vi "输入数据解析.vi"(0 "单个参数补充":dbl, 1 "从板号":dbl=1.0, 2 "主板二维码":string="BNET01", 3 "从板二维码":string="BNET01", 5 "主板引用":refnum<vi>, 7 "从板引用":refnum<vi>, 9 "主板选项":string="三级故障阀值", 11 "枚举":enum16{"主板", "从板"}(ring), 12 "快换":bool caption="快换写入") -> (4 "输出数组":dbl[][](array[numeric]), 6 "数组长度":dbl[](array[numeric]), 8 "循环次数":i32, 10 "命令":u32, 14 "名称":string[](array[string]), 15 "命令序号":u32[](array[numeric]))   [LabVIEW 2013] (continued)
                n681 = Build Array(w1614) -> (w1613:i32[])
              }
              frame 12 {
                # "SOC过高"
                n682 = Unbundle By Name(w1626) -> ("SOC过高"=w1625:dbl)
                n683 = call "输入分辨率计算-EV05.vi"("1字节?"=FALSE, "数值"=w1625, "偏移量"=0.0, "分辨率"=0.1) -> ("低字节"=w1627:dbl, "高字节1"=w1628:dbl)  [unwired: 1 in, 5 out]
                n684 = call "二进制解析-8.6.vi"("索引"=4, "数值"=w1628) -> ("低位子数组"=w1631:i32[])  [unwired: 3 out]
                n685 = call "二进制解析-8.6.vi"("索引"=4, "数值"=w1627) -> ("低位子数组"=w1623:i32[], "高位子数组"=w1630:i32[])  [unwired: 2 out]
                n686 = Insert Into Array(array=w1631, new element=w1630) -> (w1629:i32[])  [unwired: 1 in]
                n687 = call "数值二进制转十进制-8.6.vi"("子数组"=w1629) -> ("十进制数值"=w1624:i32)  [unwired: 4 out]
                n688 = disable-structure shown="启用" {
                  disable-tunnel: w1624 -> [w1639 _]
                  disable-tunnel: [w1639 255 ("高字节1")] -> w1622
                  disable-tunnel: [w1638 i32[] [] ("低位子数组 20")] -> _
                  disable-tunnel: w1623 -> [w1638 _]
                  frame Disabled {
                  }
                  frame Enabled {
                  }
                }
                n689 = Build Array(w1622, w1622) -> (w1635:i32[])
              }
              frame 13 {
                # "SOC过低"
                n690 = Unbundle By Name(w1648) -> ("SOC过低"=w1647:dbl)
                n691 = call "输入分辨率计算-EV05.vi"("1字节?"=FALSE, "数值"=w1647, "偏移量"=0.0, "分辨率"=0.1) -> ("低字节"=w1645:dbl, "高字节1"=w1646:dbl)  [unwired: 1 in, 5 out]
                n692 = call "二进制解析-8.6.vi"("索引"=4, "数值"=w1646) -> ("低位子数组"=w1643:i32[])  [unwired: 3 out]
                n693 = disable-structure shown="启用" {
                  disable-tunnel: w1645 -> [w1655 _]
                  disable-tunnel: [w1655 255 ("高字节1")] -> w1644
                  disable-tunnel: w1643 -> [w1654 _]
                  disable-tunnel: [_ 255 ("高字节1")] -> w1642
                  frame Disabled {
                    (unwired) i32[] [] ("低位子数组 4")
                  }
                  frame Enabled {
                  }
                }
                n694 = Build Array(w1642, w1644) -> (w1651:i32[])
              }
              frame 14 {
                # "内阻过大"
                n695 = disable-structure shown="启用" {
                  disable-tunnel: w1660 -> [w1665 _]
                  disable-tunnel: [w1661 255 ("高字节1")] -> w1658
                  frame Disabled {
                    n696 = Unbundle By Name(w1665) -> ("内阻过大"=w1664:dbl)
                    n697 = call "输入分辨率计算-EV05.vi"("1字节?"=TRUE, "数值"=w1664, "分辨率"=0.1) -> ("高字节1"=w1661:dbl)  [unwired: 2 in, 6 out]
                  }
                  frame Enabled {
                  }
                }
                n698 = Build Array(w1658) -> (w1659:i32[])
              }
              frame 15 {
                # "极柱温度过高"
                n699 = disable-structure shown="启用" {
                  disable-tunnel: w1669 -> [w1675 _]
                  disable-tunnel: [w1671 255 ("高字节1")] -> w1667
                  frame Disabled {
                    n700 = Unbundle By Name(w1675) -> ("极柱温度过高"=w1674:dbl)
                    n701 = call "输入分辨率计算-EV05.vi"("1字节?"=TRUE, "数值"=w1674, "偏移量"=-40.0, "分辨率"=1.0) -> ("高字节1"=w1671:dbl)  [unwired: 1 in, 6 out]
                  }
                  frame Enabled {
                  }
                }
                n702 = Build Array(w1667) -> (w1668:i32[])
              }
              frame 16 {
                # "SOH过低"
                n703 = disable-structure shown="启用" {
                  disable-tunnel: [w1692 w1700] -> w1679
                  disable-tunnel: w1678 -> [w1689 _]
                  disable-tunnel: [w1681 w1700] -> w1677
                  frame Disabled {
                    n704 = Unbundle By Name(w1689) -> ("SOH过低"=w1688:dbl)
                    n705 = call "输入分辨率计算-EV05.vi"("1字节?"=FALSE, "数值"=w1688, "偏移量"=0.0, "分辨率"=0.1) -> ("低字节"=w1690:dbl, "高字节1"=w1691:dbl)  [unwired: 1 in, 5 out]
                    n706 = call "二进制解析-8.6.vi"("索引"=4, "数值"=w1691) -> ("低位子数组"=w1694:i32[])  [unwired: 3 out]
                    n707 = call "二进制解析-8.6.vi"("索引"=4, "数值"=w1690) -> ("低位子数组"=w1683:i32[], "高位子数组"=w1693:i32[])  [unwired: 2 out]
                    n708 = call "二进制解析-8.6.vi"("索引"=4, "数值"=0) -> ("低位子数组"=w1684:i32[])  [unwired: 3 out]
                    n709 = Insert Into Array(array=w1694, new element=w1693) -> (w1687:i32[])  [unwired: 1 in]
                    n710 = Insert Into Array(array=w1683, new element=w1684) -> (w1682:i32[])  [unwired: 1 in]
                    n711 = call "数值二进制转十进制-8.6.vi"("子数组"=w1687) -> ("十进制数值"=w1692:i32)  [unwired: 4 out]
                    n712 = call "数值二进制转十进制-8.6.vi"("子数组"=w1682) -> ("十进制数值"=w1681:i32)  [unwired: 4 out]
                  }
                  frame Enabled {
                    w1700 = 255 ("高字节1")
                  }
                }
                n713 = Build Array(w1679, w1677) -> (w1680:i32[])
              }
            }
            n714 = Insert Into Array(array=w1484, new element=w1485) -> (w1483:dbl[])  [unwired: 1 in]
          }
          n715 = Build Array(w1480) -> (w1479:dbl[][])
          n716 = Build Array("一级故障阀值") -> (w1470:string[])
        }
        frame "总电压过低(2)" {
          n717 = Unbundle By Name(w1706) -> ("一级故障 2"=w1707:refnum<vi>)
          n718 = property class="Clust (严格)"(reference=w1707) -> ("Value"=w1705:T4)  [unwired: 1 in, 2 out]
          n719 = for {
            N: 17 -> [_]
            tunnel: w1705 -> [w1717]
            shift-right: [w1714] -> w1711
            shift-left: dbl[] [] -> [w1715]
            i -> [w1718]
            n720 = case shown="13" w1718 {
              tunnel: w1717 -> [w1719 w1730 w1741 w1751 w1761 w1771 w1783 w1795 w1807 w1819 w1831 w1843 w1857 w1879 w1891 w1900 w1909]
              tunnel: [w1720 w1731 w1742 w1752 w1762 w1773 w1785 w1797 w1809 w1821 w1833 w1844 w1866 w1882 w1890 w1899 w1911] -> w1716
              frame 0, Default {
                # "总电压过高"
                n721 = disable-structure shown="启用" {
                  disable-tunnel: [w1726 w1729] -> w1722
                  disable-tunnel: [w1725 w1729] -> w1721
                  disable-tunnel: w1719 -> [w1724 _]
                  frame Disabled {
                    n722 = Unbundle By Name(w1724) -> ("总电压过高"=w1723:dbl)
                    n723 = call "输入分辨率计算-EV05.vi"("1字节?"=FALSE, "数值"=w1723, "分辨率"=0.1) -> ("低字节"=w1726:dbl, "高字节1"=w1725:dbl)  [unwired: 2 in, 5 out]
                  }
                  frame Enabled {
                    w1729 = 255 ("高字节1")
                  }
                }
                n724 = Build Array(w1721, w1722) -> (w1720:i32[])
              }
              frame 1 {
                # "总电压过低"
                n725 = disable-structure shown="启用" {
                  disable-tunnel: [w1737 w1740] -> w1733
                  disable-tunnel: [w1736 w1740] -> w1732
                  disable-tunnel: w1730 -> [w1735 _]
                  frame Enabled {
                    n726 = Unbundle By Name(w1735) -> ("总电压过低"=w1734:dbl)
                    n727 = call "输入分辨率计算-EV05.vi"("1字节?"=FALSE, "数值"=w1734, "分辨率"=0.1) -> ("低字节"=w1737:dbl, "高字节1"=w1736:dbl)  [unwired: 2 in, 5 out]
                  }
                  frame Disabled {
                    w1740 = 255 ("高字节1")
                  }
                }
                n728 = Build Array(w1732, w1733) -> (w1731:dbl[])
              }
              frame 2 {
                # "温度过高"
                n729 = disable-structure shown="启用" {
                  disable-tunnel: [w1747 255 ("高字节1")] -> w1743
                  disable-tunnel: w1741 -> [w1745 _]
                  frame Disabled {
                    n730 = Unbundle By Name(w1745) -> ("温度过高"=w1744:dbl)
                    n731 = call "输入分辨率计算-EV05.vi"("1字节?"=TRUE, "数值"=w1744, "偏移量"=-40.0, "分辨率"=1.0) -> ("高字节1"=w1747:dbl)  [unwired: 1 in, 6 out]
                  }
                  frame Enabled {
                  }
                }
                n732 = Build Array(w1743) -> (w1742:i32[])
              }
              frame 3 {
                # "温度过低"
                n733 = disable-structure shown="启用" {
                  disable-tunnel: [w1757 255 ("高字节1")] -> w1753
                  disable-tunnel: w1751 -> [w1755 _]
                  frame Disabled {
                    n734 = Unbundle By Name(w1755) -> ("温度过低"=w1754:dbl)
                    n735 = call "输入分辨率计算-EV05.vi"("1字节?"=TRUE, "数值"=w1754, "偏移量"=-40.0, "分辨率"=1.0) -> ("高字节1"=w1757:dbl)  [unwired: 1 in, 6 out]
                  }
                  frame Enabled {
                  }
                }
                n736 = Build Array(w1753) -> (w1752:i32[])
              }
              frame 4 {
                # "整组温度不均衡"
                n737 = disable-structure shown="启用" {
                  disable-tunnel: [w1767 255 ("高字节1")] -> w1763
                  disable-tunnel: w1761 -> [w1765 _]
                  frame Disabled {
                    n738 = Unbundle By Name(w1765) -> ("整组温度不均衡"=w1764:dbl)
                    n739 = call "输入分辨率计算-EV05.vi"("1字节?"=TRUE, "数值"=w1764, "偏移量"=0.0, "分辨率"=1.0) -> ("高字节1"=w1767:dbl)  [unwired: 1 in, 6 out]
                  }
                  frame Enabled {
                  }
                }
                n740 = Build Array(w1763) -> (w1762:i32[])
              }
              frame 5 {
                # "单组电压不均衡"
                n741 = disable-structure shown="启用" {
                  disable-tunnel: [w1779 w1782] -> w1774
                  disable-tunnel: [w1777 w1782] -> w1772
                  disable-tunnel: w1771 -> [w1776 _]
                  frame Disabled {
                    n742 = Unbundle By Name(w1776) -> ("单组电压不均衡"=w1775:dbl)
                    n743 = call "输入分辨率计算-EV05.vi"("1字节?"=FALSE, "数值"=w1775, "偏移量"=0.0, "分辨率"=0.001) -> ("低字节"=w1777:dbl, "高字节1"=w1779:dbl)  [unwired: 1 in, 5 out]
                  }
                  frame Enabled {
                    w1782 = 255 ("高字节1")
                  }
                }
                n744 = Build Array(w1774, w1772) -> (w1773:i32[])
              }
              frame 6 {
                # "整组电压不均衡"
                n745 = disable-structure shown="启用" {
                  disable-tunnel: [w1791 w1794] -> w1786
                  disable-tunnel: [w1789 w1794] -> w1784
                  disable-tunnel: w1783 -> [w1788 _]
                  frame Disabled {
                    n746 = Unbundle By Name(w1788) -> ("整组电压不均衡"=w1787:dbl)
                    n747 = call "输入分辨率计算-EV05.vi"("1字节?"=FALSE, "数值"=w1787, "偏移量"=0.0, "分辨率"=0.001) -> ("低字节"=w1789:dbl, "高字节1"=w1791:dbl)  [unwired: 1 in, 5 out]
                  }
                  frame Enabled {
                    w1794 = 255 ("高字节1")
                  }
                }
                n748 = Build Array(w1786, w1784) -> (w1785:i32[])
              }
              frame 7 {
                # "单体电压过高"
                n749 = disable-structure shown="启用" {
                  disable-tunnel: [w1803 w1806] -> w1798
                  disable-tunnel: [w1801 w1806] -> w1796
                  disable-tunnel: w1795 -> [w1800 _]
                  frame Disabled {
                    n750 = Unbundle By Name(w1800) -> ("单体电压过高"=w1799:dbl)
                    n751 = call "输入分辨率计算-EV05.vi"("1字节?"=FALSE, "数值"=w1799, "偏移量"=0.0, "分辨率"=0.001) -> ("低字节"=w1801:dbl, "高字节1"=w1803:dbl)  [unwired: 1 in, 5 out]
                  }
                  frame Enabled {
                    w1806 = 255 ("高字节1")
                  }
                }
                n752 = Build Array(w1798, w1796) -> (w1797:i32[])
              }
              frame 8 {
                # "单体电压过低"
                n753 = disable-structure shown="启用" {
                  disable-tunnel: [w1815 w1818] -> w1810
                  disable-tunnel: [w1813 w1818] -> w1808
                  disable-tunnel: w1807 -> [w1812 _]
                  frame Disabled {
                    n754 = Unbundle By Name(w1812) -> ("单体电压过低"=w1811:dbl)
                    n755 = call "输入分辨率计算-EV05.vi"("1字节?"=FALSE, "数值"=w1811, "偏移量"=0.0, "分辨率"=0.001) -> ("低字节"=w1813:dbl, "高字节1"=w1815:dbl)  [unwired: 1 in, 5 out]
                  }
                  frame Enabled {
                    w1818 = 255 ("高字节1")
                  }
                }
                n756 = Build Array(w1810, w1808) -> (w1809:i32[])
              }
              frame 9 {
                # "充电电流过高"
                n757 = disable-structure shown="启用" {
                  disable-tunnel: [w1827 w1830] -> w1822
                  disable-tunnel: [w1825 w1830] -> w1820
                  disable-tunnel: w1819 -> [w1824 _]
                  frame Disabled {
                    n758 = Unbundle By Name(w1824) -> ("充电电流过高"=w1823:dbl)
                    n759 = call "输入分辨率计算-EV05.vi"("1字节?"=FALSE, "数值"=w1823, "偏移量"=-3000.0, "分辨率"=0.1) -> ("低字节"=w1825:dbl, "高字节1"=w1827:dbl)  [unwired: 1 in, 5 out]
                  }
                  frame Enabled {
                    w1830 = 255 ("高字节1")
                  }
                }
                n760 = Build Array(w1822, w1820) -> (w1821:i32[])
              }
              frame 10 {
                # "放电电流过高"
                n761 = disable-structure shown="启用" {
                  disable-tunnel: [w1839 w1842] -> w1834
                  disable-tunnel: [w1837 w1842] -> w1832
                  disable-tunnel: w1831 -> [w1836 _]
                  frame Disabled {
                    n762 = Unbundle By Name(w1836) -> ("放电电流过高"=w1835:dbl)
                    n763 = call "输入分辨率计算-EV05.vi"("1字节?"=FALSE, "数值"=w1835, "偏移量"=-3000.0, "分辨率"=0.1) -> ("低字节"=w1837:dbl, "高字节1"=w1839:dbl)  [unwired: 1 in, 5 out]
                  }
                  frame Enabled {
                    w1842 = 255 ("高字节1")
                  }
                }
                n764 = Build Array(w1834, w1832) -> (w1833:i32[])
              }
              frame 11 {
                # "单组温度不均衡"
                n765 = disable-structure shown="启用" {
                  disable-tunnel: [w1849 255 ("高字节1")] -> w1845
                  disable-tunnel: w1843 -> [w1847 _]
                  frame Disabled {
                    n766 = Unbundle By Name(w1847) -> ("单组温度不均衡"=w1846:dbl)
                    n767 = call "输入分辨率计算-EV05.vi"("1字节?"=TRUE, "数值"=w1846, "偏移量"=0.0, "分辨率"=1.0) -> ("高字节1"=w1849:dbl)  [unwired: 1 in, 6 out]
                  }
                  frame Enabled {
                  }
                }
                n768 = Build Array(w1845) -> (w1844:i32[])
              }
              frame 12 {
                # "SOC过高"
                n769 = Unbundle By Name(w1857) -> ("SOC过高"=w1856:dbl)
                n770 = call "输入分辨率计算-EV05.vi"("1字节?"=FALSE, "数值"=w1856, "偏移量"=0.0, "分辨率"=0.1) -> ("低字节"=w1858:dbl, "高字节1"=w1859:dbl)  [unwired: 1 in, 5 out]
                n771 = call "二进制解析-8.6.vi"("索引"=4, "数值"=w1859) -> ("低位子数组"=w1862:i32[])  [unwired: 3 out]
                n772 = call "二进制解析-8.6.vi"("索引"=4, "数值"=w1858) -> ("低位子数组"=w1854:i32[], "高位子数组"=w1861:i32[])  [unwired: 2 out]
                n773 = Insert Into Array(array=w1862, new element=w1861) -> (w1860:i32[])  [unwired: 1 in]
                n774 = call "数值二进制转十进制-8.6.vi"("子数组"=w1860) -> ("十进制数值"=w1855:i32)  [unwired: 4 out]
                n775 = disable-structure shown="启用" {
                  disable-tunnel: w1855 -> [w1870 _]
                  disable-tunnel: [w1870 255 ("高字节1")] -> w1853
                  disable-tunnel: [w1869 i32[] [] ("低位子数组 20")] -> _
                  disable-tunnel: w1854 -> [w1869 _]
                  frame Disabled {
                  }
                  frame Enabled {
                  }
                }
                n776 = Build Array(w1853, w1853) -> (w1866:i32[])
              }
              frame 13 {
                # "SOC过低"
                n777 = Unbundle By Name(w1879) -> ("SOC过低"=w1878:dbl)
                n778 = call "输入分辨率计算-EV05.vi"("1字节?"=FALSE, "数值"=w1878, "偏移量"=0.0, "分辨率"=0.1) -> ("低字节"=w1876:dbl, "高字节1"=w1877:dbl)  [unwired: 1 in, 5 out]
                n779 = call "二进制解析-8.6.vi"("索引"=4, "数值"=w1877) -> ("低位子数组"=w1874:i32[])  [unwired: 3 out]
                n780 = disable-structure shown="启用" {
                  disable-tunnel: w1876 -> [w1886 _]
                  disable-tunnel: [w1886 255 ("高字节1")] -> w1875
                  disable-tunnel: w1874 -> [w1885 _]
                  disable-tunnel: [_ 255 ("高字节1")] -> w1873
                  frame Disabled {
                    (unwired) i32[] [] ("低位子数组 4")
                  }
                  frame Enabled {
                  }
                }
                n781 = Build Array(w1873, w1875) -> (w1882:i32[])
              }
              frame 14 {
                # "内阻过大"
                n782 = disable-structure shown="启用" {
                  disable-tunnel: w1891 -> [w1896 _]
                  disable-tunnel: [w1892 255 ("高字节1")] -> w1889
                  frame Disabled {
                    n783 = Unbundle By Name(w1896) -> ("内阻过大"=w1895:dbl)
                    n784 = call "输入分辨率计算-EV05.vi"("1字节?"=TRUE, "数值"=w1895, "分辨率"=0.1) -> ("高字节1"=w1892:dbl)  [unwired: 2 in, 6 out]
                  }
                  frame Enabled {
                  }
                }
                n785 = Build Array(w1889) -> (w1890:i32[])
              }
              frame 15 {
                # "极柱温度过高"
                n786 = disable-structure shown="启用" {
                  disable-tunnel: w1900 -> [w1906 _]
                  disable-tunnel: [w1902 255 ("高字节1")] -> w1898
                  frame Disabled {
                    n787 = Unbundle By Name(w1906) -> ("极柱温度过高"=w1905:dbl)
                    n788 = call "输入分辨率计算-EV05.vi"("1字节?"=TRUE, "数值"=w1905, "偏移量"=-40.0, "分辨率"=1.0) -> ("高字节1"=w1902:dbl)  [unwired: 1 in, 6 out]
                  }
                  frame Enabled {
                  }
                }
                n789 = Build Array(w1898) -> (w1899:i32[])
              }
              frame 16 {
                # "SOH过低"
                n790 = disable-structure shown="启用" {
                  disable-tunnel: [w1923 w1931] -> w1910
                  disable-tunnel: w1909 -> [w1920 _]
                  disable-tunnel: [w1912 w1931] -> w1908
                  frame Disabled {
                    n791 = Unbundle By Name(w1920) -> ("SOH过低"=w1919:dbl)
                    n792 = call "输入分辨率计算-EV05.vi"("1字节?"=FALSE, "数值"=w1919, "偏移量"=0.0, "分辨率"=0.1) -> ("低字节"=w1921:dbl, "高字节1"=w1922:dbl)  [unwired: 1 in, 5 out]
                    n793 = call "二进制解析-8.6.vi"("索引"=4, "数值"=w1922) -> ("低位子数组"=w1925:i32[])  [unwired: 3 out]
                    n794 = call "二进制解析-8.6.vi"("索引"=4, "数值"=w1921) -> ("低位子数组"=w1914:i32[], "高位子数组"=w1924:i32[])  [unwired: 2 out]
                    n795 = call "二进制解析-8.6.vi"("索引"=4, "数值"=0) -> ("低位子数组"=w1915:i32[])  [unwired: 3 out]
                    n796 = Insert Into Array(array=w1925, new element=w1924) -> (w1918:i32[])  [unwired: 1 in]
                    n797 = Insert Into Array(array=w1914, new element=w1915) -> (w1913:i32[])  [unwired: 1 in]
                    n798 = call "数值二进制转十进制-8.6.vi"("子数组"=w1918) -> ("十进制数值"=w1923:i32)  [unwired: 4 out]
                    n799 = call "数值二进制转十进制-8.6.vi"("子数组"=w1913) -> ("十进制数值"=w1912:i32)  [unwired: 4 out]
                  }
                  frame Enabled {
                    w1931 = 255 ("高字节1")
                  }
                }
                n800 = Build Array(w1910, w1908) -> (w1911:i32[])
              }
            }
            n801 = Insert Into Array(array=w1715, new element=w1716) -> (w1714:dbl[])  [unwired: 1 in]
          }
          n802 = Build Array(w1711) -> (w1710:dbl[][])
          n803 = Build Array("二级故障阀值") -> (w1701:string[])
        }
        frame "总电压过低(3)" {
          n804 = Unbundle By Name(w1937) -> ("一级故障 3"=w1938:refnum<vi>)
          n805 = property class="Clust (严格)"(reference=w1938) -> ("Value"=w1936:T4)  [unwired: 1 in, 2 out]
          n806 = for {
            N: 17 -> [_]
            tunnel: w1936 -> [w1948]
            shift-right: [w1945] -> w1942
            shift-left: dbl[] [] -> [w1946]
            i -> [w1949]
            n807 = case shown="13" w1949 {
              tunnel: w1948 -> [w1950 w1961 w1972 w1982 w1992 w2002 w2014 w2026 w2038 w2050 w2062 w2074 w2088 w2110 w2122 w2131 w2140]
              tunnel: [w1951 w1962 w1973 w1983 w1993 w2004 w2016 w2028 w2040 w2052 w2064 w2075 w2097 w2113 w2121 w2130 w2142] -> w1947
              frame 0, Default {
                # "总电压过高"
                n808 = disable-structure shown="启用" {
                  disable-tunnel: [w1957 w1960] -> w1953
                  disable-tunnel: [w1956 w1960] -> w1952
                  disable-tunnel: w1950 -> [w1955 _]
                  frame Disabled {
                    n809 = Unbundle By Name(w1955) -> ("总电压过高"=w1954:dbl)
                    n810 = call "输入分辨率计算-EV05.vi"("1字节?"=FALSE, "数值"=w1954, "分辨率"=0.1) -> ("低字节"=w1957:dbl, "高字节1"=w1956:dbl)  [unwired: 2 in, 5 out]
                  }
                  frame Enabled {
                    w1960 = 255 ("高字节1")
                  }
                }
                n811 = Build Array(w1952, w1953) -> (w1951:i32[])
              }
              frame 1 {
                # "总电压过低"
                n812 = disable-structure shown="启用" {
                  disable-tunnel: [w1968 w1971] -> w1964
                  disable-tunnel: [w1967 w1971] -> w1963
                  disable-tunnel: w1961 -> [w1966 _]
                  frame Enabled {
                    n813 = Unbundle By Name(w1966) -> ("总电压过低"=w1965:dbl)
                    n814 = call "输入分辨率计算-EV05.vi"("1字节?"=FALSE, "数值"=w1965, "分辨率"=0.1) -> ("低字节"=w1968:dbl, "高字节1"=w1967:dbl)  [unwired: 2 in, 5 out]
                  }
                  frame Disabled {
                    w1971 = 255 ("高字节1")
                  }
                }
                n815 = Build Array(w1963, w1964) -> (w1962:dbl[])
              }
              frame 2 {
                # "温度过高"
                n816 = disable-structure shown="启用" {
                  disable-tunnel: [w1978 255 ("高字节1")] -> w1974
                  disable-tunnel: w1972 -> [w1976 _]
                  frame Disabled {
                    n817 = Unbundle By Name(w1976) -> ("温度过高"=w1975:dbl)
                    n818 = call "输入分辨率计算-EV05.vi"("1字节?"=TRUE, "数值"=w1975, "偏移量"=-40.0, "分辨率"=1.0) -> ("高字节1"=w1978:dbl)  [unwired: 1 in, 6 out]
                  }
                  frame Enabled {
                  }
                }
                n819 = Build Array(w1974) -> (w1973:i32[])
              }
              frame 3 {
                # "温度过低"
                n820 = disable-structure shown="启用" {
                  disable-tunnel: [w1988 255 ("高字节1")] -> w1984
                  disable-tunnel: w1982 -> [w1986 _]
                  frame Disabled {
                    n821 = Unbundle By Name(w1986) -> ("温度过低"=w1985:dbl)
                    n822 = call "输入分辨率计算-EV05.vi"("1字节?"=TRUE, "数值"=w1985, "偏移量"=-40.0, "分辨率"=1.0) -> ("高字节1"=w1988:dbl)  [unwired: 1 in, 6 out]
                  }
                  frame Enabled {
                  }
                }
                n823 = Build Array(w1984) -> (w1983:i32[])
              }
              frame 4 {
                # "整组温度不均衡"
                n824 = disable-structure shown="启用" {
                  disable-tunnel: [w1998 255 ("高字节1")] -> w1994
                  disable-tunnel: w1992 -> [w1996 _]
                  frame Disabled {
                    n825 = Unbundle By Name(w1996) -> ("整组温度不均衡"=w1995:dbl)
                    n826 = call "输入分辨率计算-EV05.vi"("1字节?"=TRUE, "数值"=w1995, "偏移量"=0.0, "分辨率"=1.0) -> ("高字节1"=w1998:dbl)  [unwired: 1 in, 6 out]
                  }
                  frame Enabled {
                  }
                }
                n827 = Build Array(w1994) -> (w1993:i32[])
              }
              frame 5 {
                # "单组电压不均衡"
                n828 = disable-structure shown="启用" {
                  disable-tunnel: [w2010 w2013] -> w2005
                  disable-tunnel: [w2008 w2013] -> w2003
                  disable-tunnel: w2002 -> [w2007 _]
                  frame Disabled {
                    n829 = Unbundle By Name(w2007) -> ("单组电压不均衡"=w2006:dbl)
                    n830 = call "输入分辨率计算-EV05.vi"("1字节?"=FALSE, "数值"=w2006, "偏移量"=0.0, "分辨率"=0.001) -> ("低字节"=w2008:dbl, "高字节1"=w2010:dbl)  [unwired: 1 in, 5 out]
                  }
                  frame Enabled {
                    w2013 = 255 ("高字节1")
                  }
                }
                n831 = Build Array(w2005, w2003) -> (w2004:i32[])
              }
              frame 6 {
                # "整组电压不均衡"
                n832 = disable-structure shown="启用" {
                  disable-tunnel: [w2022 w2025] -> w2017
                  disable-tunnel: [w2020 w2025] -> w2015
                  disable-tunnel: w2014 -> [w2019 _]
                  frame Disabled {
                    n833 = Unbundle By Name(w2019) -> ("整组电压不均衡"=w2018:dbl)
                    n834 = call "输入分辨率计算-EV05.vi"("1字节?"=FALSE, "数值"=w2018, "偏移量"=0.0, "分辨率"=0.001) -> ("低字节"=w2020:dbl, "高字节1"=w2022:dbl)  [unwired: 1 in, 5 out]
                  }
                  frame Enabled {
                    w2025 = 255 ("高字节1")
                  }
                }
                n835 = Build Array(w2017, w2015) -> (w2016:i32[])
              }
              frame 7 {
                # "单体电压过高"
                n836 = disable-structure shown="启用" {
                  disable-tunnel: [w2034 w2037] -> w2029
                  disable-tunnel: [w2032 w2037] -> w2027
                  disable-tunnel: w2026 -> [w2031 _]
                  frame Disabled {
                    n837 = Unbundle By Name(w2031) -> ("单体电压过高"=w2030:dbl)
                    n838 = call "输入分辨率计算-EV05.vi"("1字节?"=FALSE, "数值"=w2030, "偏移量"=0.0, "分辨率"=0.001) -> ("低字节"=w2032:dbl, "高字节1"=w2034:dbl)  [unwired: 1 in, 5 out]
                  }
                  frame Enabled {
                    w2037 = 255 ("高字节1")
                  }
                }
                n839 = Build Array(w2029, w2027) -> (w2028:i32[])
              }
              frame 8 {
                # "单体电压过低"
                n840 = disable-structure shown="启用" {
                  disable-tunnel: [w2046 w2049] -> w2041
                  disable-tunnel: [w2044 w2049] -> w2039
                  disable-tunnel: w2038 -> [w2043 _]
                  frame Disabled {
                    n841 = Unbundle By Name(w2043) -> ("单体电压过低"=w2042:dbl)
                    n842 = call "输入分辨率计算-EV05.vi"("1字节?"=FALSE, "数值"=w2042, "偏移量"=0.0, "分辨率"=0.001) -> ("低字节"=w2044:dbl, "高字节1"=w2046:dbl)  [unwired: 1 in, 5 out]
                  }
                  frame Enabled {
                    w2049 = 255 ("高字节1")
                  }
                }
                n843 = Build Array(w2041, w2039) -> (w2040:i32[])
              }
              frame 9 {
                # "充电电流过高"
                n844 = disable-structure shown="启用" {
                  disable-tunnel: [w2058 w2061] -> w2053
                  disable-tunnel: [w2056 w2061] -> w2051
                  disable-tunnel: w2050 -> [w2055 _]
                  frame Disabled {
                    n845 = Unbundle By Name(w2055) -> ("充电电流过高"=w2054:dbl)
                    n846 = call "输入分辨率计算-EV05.vi"("1字节?"=FALSE, "数值"=w2054, "偏移量"=-3000.0, "分辨率"=0.1) -> ("低字节"=w2056:dbl, "高字节1"=w2058:dbl)  [unwired: 1 in, 5 out]
                  }
                  frame Enabled {
                    w2061 = 255 ("高字节1")
                  }
                }
                n847 = Build Array(w2053, w2051) -> (w2052:i32[])
              }
              frame 10 {
                # "放电电流过高"
                n848 = disable-structure shown="启用" {
                  disable-tunnel: [w2070 w2073] -> w2065
                  disable-tunnel: [w2068 w2073] -> w2063
                  disable-tunnel: w2062 -> [w2067 _]
                  frame Disabled {
                    n849 = Unbundle By Name(w2067) -> ("放电电流过高"=w2066:dbl)
                    n850 = call "输入分辨率计算-EV05.vi"("1字节?"=FALSE, "数值"=w2066, "偏移量"=-3000.0, "分辨率"=0.1) -> ("低字节"=w2068:dbl, "高字节1"=w2070:dbl)  [unwired: 1 in, 5 out]
                  }
                  frame Enabled {
                    w2073 = 255 ("高字节1")
                  }
                }
                n851 = Build Array(w2065, w2063) -> (w2064:i32[])
              }
              frame 11 {
                # "单组温度不均衡"
                n852 = disable-structure shown="启用" {
                  disable-tunnel: [w2080 255 ("高字节1")] -> w2076
                  disable-tunnel: w2074 -> [w2078 _]
                  frame Disabled {
                    n853 = Unbundle By Name(w2078) -> ("单组温度不均衡"=w2077:dbl)
                    n854 = call "输入分辨率计算-EV05.vi"("1字节?"=TRUE, "数值"=w2077, "偏移量"=0.0, "分辨率"=1.0) -> ("高字节1"=w2080:dbl)  [unwired: 1 in, 6 out]
                  }
                  frame Enabled {
                  }
                }
                n855 = Build Array(w2076) -> (w2075:i32[])
              }
              frame 12 {
                # "SOC过高"
                n856 = Unbundle By Name(w2088) -> ("SOC过高"=w2087:dbl)
                n857 = call "输入分辨率计算-EV05.vi"("1字节?"=FALSE, "数值"=w2087, "偏移量"=0.0, "分辨率"=0.1) -> ("低字节"=w2089:dbl, "高字节1"=w2090:dbl)  [unwired: 1 in, 5 out]
                n858 = call "二进制解析-8.6.vi"("索引"=4, "数值"=w2090) -> ("低位子数组"=w2093:i32[])  [unwired: 3 out]
                n859 = call "二进制解析-8.6.vi"("索引"=4, "数值"=w2089) -> ("低位子数组"=w2085:i32[], "高位子数组"=w2092:i32[])  [unwired: 2 out]
                n860 = Insert Into Array(array=w2093, new element=w2092) -> (w2091:i32[])  [unwired: 1 in]
                n861 = call "数值二进制转十进制-8.6.vi"("子数组"=w2091) -> ("十进制数值"=w2086:i32)  [unwired: 4 out]
                n862 = disable-structure shown="启用" {
                  disable-tunnel: w2086 -> [w2101 _]
                  disable-tunnel: [w2101 255 ("高字节1")] -> w2084
                  disable-tunnel: [w2100 i32[] [] ("低位子数组 20")] -> _
                  disable-tunnel: w2085 -> [w2100 _]
                  frame Disabled {
                  }
                  frame Enabled {
                  }
                }
                n863 = Build Array(w2084, w2084) -> (w2097:i32[])
              }
              frame 13 {
                # "SOC过低"
                n864 = Unbundle By Name(w2110) -> ("SOC过低"=w2109:dbl)
                n865 = call "输入分辨率计算-EV05.vi"("1字节?"=FALSE, "数值"=w2109, "偏移量"=0.0, "分辨率"=0.1) -> ("低字节"=w2107:dbl, "高字节1"=w2108:dbl)  [unwired: 1 in, 5 out]
                n866 = call "二进制解析-8.6.vi"("索引"=4, "数值"=w2108) -> ("低位子数组"=w2105:i32[])  [unwired: 3 out]
                n867 = disable-structure shown="启用" {
                  disable-tunnel: w2107 -> [w2117 _]
                  disable-tunnel: [w2117 255 ("高字节1")] -> w2106
                  disable-tunnel: w2105 -> [w2116 _]
                  disable-tunnel: [_ 255 ("高字节1")] -> w2104
                  frame Disabled {
                    (unwired) i32[] [] ("低位子数组 4")
                  }
                  frame Enabled {
                  }
                }
                n868 = Build Array(w2104, w2106) -> (w2113:i32[])
              }
              frame 14 {
                # "内阻过大"
                n869 = disable-structure shown="启用" {
                  disable-tunnel: w2122 -> [w2127 _]
                  disable-tunnel: [w2123 255 ("高字节1")] -> w2120
                  frame Disabled {
                    n870 = Unbundle By Name(w2127) -> ("内阻过大"=w2126:dbl)
                    n871 = call "输入分辨率计算-EV05.vi"("1字节?"=TRUE, "数值"=w2126, "分辨率"=0.1) -> ("高字节1"=w2123:dbl)  [unwired: 2 in, 6 out]
                  }
                  frame Enabled {
                  }
                }
                n872 = Build Array(w2120) -> (w2121:i32[])
              }
              frame 15 {
                # "极柱温度过高"
                n873 = disable-structure shown="启用" {
                  disable-tunnel: w2131 -> [w2137 _]
                  disable-tunnel: [w2133 255 ("高字节1")] -> w2129
                  frame Disabled {
                    n874 = Unbundle By Name(w2137) -> ("极柱温度过高"=w2136:dbl)
                    n875 = call "输入分辨率计算-EV05.vi"("1字节?"=TRUE, "数值"=w2136, "偏移量"=-40.0, "分辨率"=1.0) -> ("高字节1"=w2133:dbl)  [unwired: 1 in, 6 out]
                  }
                  frame Enabled {
                  }
                }
                n876 = Build Array(w2129) -> (w2130:i32[])
              }
              frame 16 {
                # "SOH过低"
                n877 = disable-structure shown="启用" {
                  disable-tunnel: [w2154 w2162] -> w2141
                  disable-tunnel: w2140 -> [w2151 _]
                  disable-tunnel: [w2143 w2162] -> w2139
                  frame Disabled {
                    n878 = Unbundle By Name(w2151) -> ("SOH过低"=w2150:dbl)
                    n879 = call "输入分辨率计算-EV05.vi"("1字节?"=FALSE, "数值"=w2150, "偏移量"=0.0, "分辨率"=0.1) -> ("低字节"=w2152:dbl, "高字节1"=w2153:dbl)  [unwired: 1 in, 5 out]
                    n880 = call "二进制解析-8.6.vi"("索引"=4, "数值"=w2153) -> ("低位子数组"=w2156:i32[])  [unwired: 3 out]
                    n881 = call "二进制解析-8.6.vi"("索引"=4, "数值"=w2152) -> ("低位子数组"=w2145:i32[], "高位子数组"=w2155:i32[])  [unwired: 2 out]
                    n882 = call "二进制解析-8.6.vi"("索引"=4, "数值"=0) -> ("低位子数组"=w2146:i32[])  [unwired: 3 out]
                    n883 = Insert Into Array(array=w2156, new element=w2155) -> (w2149:i32[])  [unwired: 1 in]
                    n884 = Insert Into Array(array=w2145, new element=w2146) -> (w2144:i32[])  [unwired: 1 in]
                    n885 = call "数值二进制转十进制-8.6.vi"("子数组"=w2149) -> ("十进制数值"=w2154:i32)  [unwired: 4 out]
                    n886 = call "数值二进制转十进制-8.6.vi"("子数组"=w2144) -> ("十进制数值"=w2143:i32)  [unwired: 4 out]
                  }
                  frame Enabled {
                    w2162 = 255 ("高字节1")
                  }
                }
                n887 = Build Array(w2141, w2139) -> (w2142:i32[])
              }
            }
            n888 = Insert Into Array(array=w1946, new element=w1947) -> (w1945:dbl[])  [unwired: 1 in]
          }
          n889 = Build Array(w1942) -> (w1941:dbl[][])
          n890 = Build Array("三级故障阀值") -> (w1932:string[])
        }
        frame "总电压过高(2)" {
          n891 = Unbundle By Name(w2168) -> ("一级故障 2"=w2169:refnum<vi>)
          n892 = property class="Clust (严格)"(reference=w2169) -> ("Value"=w2167:T4)  [unwired: 1 in, 2 out]
          n893 = for {
            N: 17 -> [_]
            tunnel: w2167 -> [w2179]
            shift-right: [w2176] -> w2173
            shift-left: dbl[] [] -> [w2177]
            i -> [w2180]
            n894 = case shown="13" w2180 {
              tunnel: w2179 -> [w2181 w2192 w2203 w2213 w2223 w2233 w2245 w2257 w2269 w2281 w2293 w2305 w2319 w2341 w2353 w2362 w2371]
              tunnel: [w2182 w2193 w2204 w2214 w2224 w2235 w2247 w2259 w2271 w2283 w2295 w2306 w2328 w2344 w2352 w2361 w2373] -> w2178
              frame 0, Default {
                # "总电压过高"
                n895 = disable-structure shown="启用" {
                  disable-tunnel: [w2188 w2191] -> w2184
                  disable-tunnel: [w2187 w2191] -> w2183
                  disable-tunnel: w2181 -> [w2186 _]
                  frame Enabled {
                    n896 = Unbundle By Name(w2186) -> ("总电压过高"=w2185:dbl)
                    n897 = call "输入分辨率计算-EV05.vi"("1字节?"=FALSE, "数值"=w2185, "分辨率"=0.1) -> ("低字节"=w2188:dbl, "高字节1"=w2187:dbl)  [unwired: 2 in, 5 out]
                  }
                  frame Disabled {
                    w2191 = 255 ("高字节1")
                  }
                }
                n898 = Build Array(w2183, w2184) -> (w2182:dbl[])
              }
              frame 1 {
                # "总电压过低"
                n899 = disable-structure shown="启用" {
                  disable-tunnel: [w2199 w2202] -> w2195
                  disable-tunnel: [w2198 w2202] -> w2194
                  disable-tunnel: w2192 -> [w2197 _]
                  frame Disabled {
                    n900 = Unbundle By Name(w2197) -> ("总电压过低"=w2196:dbl)
                    n901 = call "输入分辨率计算-EV05.vi"("1字节?"=FALSE, "数值"=w2196, "分辨率"=0.1) -> ("低字节"=w2199:dbl, "高字节1"=w2198:dbl)  [unwired: 2 in, 5 out]
                  }
                  frame Enabled {
                    w2202 = 255 ("高字节1")
                  }
                }
                n902 = Build Array(w2194, w2195) -> (w2193:i32[])
              }
              frame 2 {
                # "温度过高"
                n903 = disable-structure shown="启用" {
                  disable-tunnel: [w2209 255 ("高字节1")] -> w2205
                  disable-tunnel: w2203 -> [w2207 _]
                  frame Disabled {
                    n904 = Unbundle By Name(w2207) -> ("温度过高"=w2206:dbl)
                    n905 = call "输入分辨率计算-EV05.vi"("1字节?"=TRUE, "数值"=w2206, "偏移量"=-40.0, "分辨率"=1.0) -> ("高字节1"=w2209:dbl)  [unwired: 1 in, 6 out]
                  }
                  frame Enabled {
                  }
                }
                n906 = Build Array(w2205) -> (w2204:i32[])
              }
              frame 3 {
                # "温度过低"
                n907 = disable-structure shown="启用" {
                  disable-tunnel: [w2219 255 ("高字节1")] -> w2215
                  disable-tunnel: w2213 -> [w2217 _]
                  frame Disabled {
                    n908 = Unbundle By Name(w2217) -> ("温度过低"=w2216:dbl)
                    n909 = call "输入分辨率计算-EV05.vi"("1字节?"=TRUE, "数值"=w2216, "偏移量"=-40.0, "分辨率"=1.0) -> ("高字节1"=w2219:dbl)  [unwired: 1 in, 6 out]
                  }
                  frame Enabled {
                  }
                }
                n910 = Build Array(w2215) -> (w2214:i32[])
              }
              frame 4 {
                # "整组温度不均衡"
                n911 = disable-structure shown="启用" {
                  disable-tunnel: [w2229 255 ("高字节1")] -> w2225
                  disable-tunnel: w2223 -> [w2227 _]
                  frame Disabled {
                    n912 = Unbundle By Name(w2227) -> ("整组温度不均衡"=w2226:dbl)
                    n913 = call "输入分辨率计算-EV05.vi"("1字节?"=TRUE, "数值"=w2226, "偏移量"=0.0, "分辨率"=1.0) -> ("高字节1"=w2229:dbl)  [unwired: 1 in, 6 out]
                  }
                  frame Enabled {
                  }
                }
                n914 = Build Array(w2225) -> (w2224:i32[])
              }
              frame 5 {
                # "单组电压不均衡"
                n915 = disable-structure shown="启用" {
                  disable-tunnel: [w2241 w2244] -> w2236
                  disable-tunnel: [w2239 w2244] -> w2234
                  disable-tunnel: w2233 -> [w2238 _]
                  frame Disabled {
                    n916 = Unbundle By Name(w2238) -> ("单组电压不均衡"=w2237:dbl)
                    n917 = call "输入分辨率计算-EV05.vi"("1字节?"=FALSE, "数值"=w2237, "偏移量"=0.0, "分辨率"=0.001) -> ("低字节"=w2239:dbl, "高字节1"=w2241:dbl)  [unwired: 1 in, 5 out]
                  }
                  frame Enabled {
                    w2244 = 255 ("高字节1")
                  }
                }
                n918 = Build Array(w2236, w2234) -> (w2235:i32[])
              }
              frame 6 {
                # "整组电压不均衡"
                n919 = disable-structure shown="启用" {
                  disable-tunnel: [w2253 w2256] -> w2248
                  disable-tunnel: [w2251 w2256] -> w2246
                  disable-tunnel: w2245 -> [w2250 _]
                  frame Disabled {
                    n920 = Unbundle By Name(w2250) -> ("整组电压不均衡"=w2249:dbl)
                    n921 = call "输入分辨率计算-EV05.vi"("1字节?"=FALSE, "数值"=w2249, "偏移量"=0.0, "分辨率"=0.001) -> ("低字节"=w2251:dbl, "高字节1"=w2253:dbl)  [unwired: 1 in, 5 out]
                  }
                  frame Enabled {
                    w2256 = 255 ("高字节1")
                  }
                }
                n922 = Build Array(w2248, w2246) -> (w2247:i32[])
              }
              frame 7 {
                # "单体电压过高"
                n923 = disable-structure shown="启用" {
                  disable-tunnel: [w2265 w2268] -> w2260
                  disable-tunnel: [w2263 w2268] -> w2258
                  disable-tunnel: w2257 -> [w2262 _]
                  frame Disabled {
                    n924 = Unbundle By Name(w2262) -> ("单体电压过高"=w2261:dbl)
                    n925 = call "输入分辨率计算-EV05.vi"("1字节?"=FALSE, "数值"=w2261, "偏移量"=0.0, "分辨率"=0.001) -> ("低字节"=w2263:dbl, "高字节1"=w2265:dbl)  [unwired: 1 in, 5 out]
                  }
                  frame Enabled {
                    w2268 = 255 ("高字节1")
                  }
                }
                n926 = Build Array(w2260, w2258) -> (w2259:i32[])
              }
              frame 8 {
                # "单体电压过低"
                n927 = disable-structure shown="启用" {
                  disable-tunnel: [w2277 w2280] -> w2272
                  disable-tunnel: [w2275 w2280] -> w2270
                  disable-tunnel: w2269 -> [w2274 _]
                  frame Disabled {
                    n928 = Unbundle By Name(w2274) -> ("单体电压过低"=w2273:dbl)
                    n929 = call "输入分辨率计算-EV05.vi"("1字节?"=FALSE, "数值"=w2273, "偏移量"=0.0, "分辨率"=0.001) -> ("低字节"=w2275:dbl, "高字节1"=w2277:dbl)  [unwired: 1 in, 5 out]
                  }
                  frame Enabled {
                    w2280 = 255 ("高字节1")
                  }
                }
                n930 = Build Array(w2272, w2270) -> (w2271:i32[])
              }
              frame 9 {
                # "充电电流过高"
                n931 = disable-structure shown="启用" {
                  disable-tunnel: [w2289 w2292] -> w2284
                  disable-tunnel: [w2287 w2292] -> w2282
                  disable-tunnel: w2281 -> [w2286 _]
                  frame Disabled {
                    n932 = Unbundle By Name(w2286) -> ("充电电流过高"=w2285:dbl)
                    n933 = call "输入分辨率计算-EV05.vi"("1字节?"=FALSE, "数值"=w2285, "偏移量"=-3000.0, "分辨率"=0.1) -> ("低字节"=w2287:dbl, "高字节1"=w2289:dbl)  [unwired: 1 in, 5 out]
                  }
                  frame Enabled {
                    w2292 = 255 ("高字节1")
                  }
                }
                n934 = Build Array(w2284, w2282) -> (w2283:i32[])
              }
              frame 10 {
                # "放电电流过高"
                n935 = disable-structure shown="启用" {
                  disable-tunnel: [w2301 w2304] -> w2296
                  disable-tunnel: [w2299 w2304] -> w2294
                  disable-tunnel: w2293 -> [w2298 _]
                  frame Disabled {
                    n936 = Unbundle By Name(w2298) -> ("放电电流过高"=w2297:dbl)
                    n937 = call "输入分辨率计算-EV05.vi"("1字节?"=FALSE, "数值"=w2297, "偏移量"=-3000.0, "分辨率"=0.1) -> ("低字节"=w2299:dbl, "高字节1"=w2301:dbl)  [unwired: 1 in, 5 out]
                  }
                  frame Enabled {
                    w2304 = 255 ("高字节1")
                  }
                }
                n938 = Build Array(w2296, w2294) -> (w2295:i32[])
              }
              frame 11 {
                # "单组温度不均衡"
                n939 = disable-structure shown="启用" {
                  disable-tunnel: [w2311 255 ("高字节1")] -> w2307
                  disable-tunnel: w2305 -> [w2309 _]
                  frame Disabled {
                    n940 = Unbundle By Name(w2309) -> ("单组温度不均衡"=w2308:dbl)
                    n941 = call "输入分辨率计算-EV05.vi"("1字节?"=TRUE, "数值"=w2308, "偏移量"=0.0, "分辨率"=1.0) -> ("高字节1"=w2311:dbl)  [unwired: 1 in, 6 out]
                  }
                  frame Enabled {
                  }
                }
                n942 = Build Array(w2307) -> (w2306:i32[])
              }
              frame 12 {
                # "SOC过高"
                n943 = Unbundle By Name(w2319) -> ("SOC过高"=w2318:dbl)
                n944 = call "输入分辨率计算-EV05.vi"("1字节?"=FALSE, "数值"=w2318, "偏移量"=0.0, "分辨率"=0.1) -> ("低字节"=w2320:dbl, "高字节1"=w2321:dbl)  [unwired: 1 in, 5 out]
                n945 = call "二进制解析-8.6.vi"("索引"=4, "数值"=w2321) -> ("低位子数组"=w2324:i32[])  [unwired: 3 out]
                n946 = call "二进制解析-8.6.vi"("索引"=4, "数值"=w2320) -> ("低位子数组"=w2316:i32[], "高位子数组"=w2323:i32[])  [unwired: 2 out]
                n947 = Insert Into Array(array=w2324, new element=w2323) -> (w2322:i32[])  [unwired: 1 in]
                n948 = call "数值二进制转十进制-8.6.vi"("子数组"=w2322) -> ("十进制数值"=w2317:i32)  [unwired: 4 out]
                n949 = disable-structure shown="启用" {
                  disable-tunnel: w2317 -> [w2332 _]
                  disable-tunnel: [w2332 255 ("高字节1")] -> w2315
                  disable-tunnel: [w2331 i32[] [] ("低位子数组 20")] -> _
                  disable-tunnel: w2316 -> [w2331 _]
                  frame Disabled {
                  }
                  frame Enabled {
                  }
                }
                n950 = Build Array(w2315, w2315) -> (w2328:i32[])
              }
              frame 13 {
                # "SOC过低"
                n951 = Unbundle By Name(w2341) -> ("SOC过低"=w2340:dbl)
                n952 = call "输入分辨率计算-EV05.vi"("1字节?"=FALSE, "数值"=w2340, "偏移量"=0.0, "分辨率"=0.1) -> ("低字节"=w2338:dbl, "高字节1"=w2339:dbl)  [unwired: 1 in, 5 out]
                n953 = call "二进制解析-8.6.vi"("索引"=4, "数值"=w2339) -> ("低位子数组"=w2336:i32[])  [unwired: 3 out]
                n954 = disable-structure shown="启用" {
                  disable-tunnel: w2338 -> [w2348 _]
                  disable-tunnel: [w2348 255 ("高字节1")] -> w2337
                  disable-tunnel: w2336 -> [w2347 _]
                  disable-tunnel: [_ 255 ("高字节1")] -> w2335
                  frame Disabled {
                    (unwired) i32[] [] ("低位子数组 4")
                  }
                  frame Enabled {
                  }
                }
                n955 = Build Array(w2335, w2337) -> (w2344:i32[])
              }
              frame 14 {
                # "内阻过大"
                n956 = disable-structure shown="启用" {
                  disable-tunnel: w2353 -> [w2358 _]
                  disable-tunnel: [w2354 255 ("高字节1")] -> w2351
                  frame Disabled {
                    n957 = Unbundle By Name(w2358) -> ("内阻过大"=w2357:dbl)
                    n958 = call "输入分辨率计算-EV05.vi"("1字节?"=TRUE, "数值"=w2357, "分辨率"=0.1) -> ("高字节1"=w2354:dbl)  [unwired: 2 in, 6 out]
                  }
                  frame Enabled {
                  }
                }
                n959 = Build Array(w2351) -> (w2352:i32[])
              }
              frame 15 {
                # "极柱温度过高"
                n960 = disable-structure shown="启用" {
                  disable-tunnel: w2362 -> [w2368 _]
                  disable-tunnel: [w2364 255 ("高字节1")] -> w2360
                  frame Disabled {
                    n961 = Unbundle By Name(w2368) -> ("极柱温度过高"=w2367:dbl)
                    n962 = call "输入分辨率计算-EV05.vi"("1字节?"=TRUE, "数值"=w2367, "偏移量"=-40.0, "分辨率"=1.0) -> ("高字节1"=w2364:dbl)  [unwired: 1 in, 6 out]
                  }
                  frame Enabled {
                  }
                }
                n963 = Build Array(w2360) -> (w2361:i32[])
              }
              frame 16 {
                # "SOH过低"
                n964 = disable-structure shown="启用" {
                  disable-tunnel: [w2385 w2393] -> w2372
                  disable-tunnel: w2371 -> [w2382 _]
                  disable-tunnel: [w2374 w2393] -> w2370
                  frame Disabled {
                    n965 = Unbundle By Name(w2382) -> ("SOH过低"=w2381:dbl)
                    n966 = call "输入分辨率计算-EV05.vi"("1字节?"=FALSE, "数值"=w2381, "偏移量"=0.0, "分辨率"=0.1) -> ("低字节"=w2383:dbl, "高字节1"=w2384:dbl)  [unwired: 1 in, 5 out]
                    n967 = call "二进制解析-8.6.vi"("索引"=4, "数值"=w2384) -> ("低位子数组"=w2387:i32[])  [unwired: 3 out]
                    n968 = call "二进制解析-8.6.vi"("索引"=4, "数值"=w2383) -> ("低位子数组"=w2376:i32[], "高位子数组"=w2386:i32[])  [unwired: 2 out]
                    n969 = call "二进制解析-8.6.vi"("索引"=4, "数值"=0) -> ("低位子数组"=w2377:i32[])  [unwired: 3 out]
                    n970 = Insert Into Array(array=w2387, new element=w2386) -> (w2380:i32[])  [unwired: 1 in]
                    n971 = Insert Into Array(array=w2376, new element=w2377) -> (w2375:i32[])  [unwired: 1 in]
                    n972 = call "数值二进制转十进制-8.6.vi"("子数组"=w2380) -> ("十进制数值"=w2385:i32)  [unwired: 4 out]
                    n973 = call "数值二进制转十进制-8.6.vi"("子数组"=w2375) -> ("十进制数值"=w2374:i32)  [unwired: 4 out]
                  }
                  frame Enabled {
                    w2393 = 255 ("高字节1")
                  }
                }
                n974 = Build Array(w2372, w2370) -> (w2373:i32[])
              }
            }
            n975 = Insert Into Array(array=w2177, new element=w2178) -> (w2176:dbl[])  [unwired: 1 in]
          }
          n976 = Build Array(w2173) -> (w2172:dbl[][])
          n977 = Build Array("二级故障阀值") -> (w2163:string[])
        }
        frame "总电压过高(3)" {
          n978 = Unbundle By Name(w2399) -> ("一级故障 3"=w2400:refnum<vi>)
          n979 = property class="Clust (严格)"(reference=w2400) -> ("Value"=w2398:T4)  [unwired: 1 in, 2 out]
          n980 = for {
            N: 17 -> [_]
            tunnel: w2398 -> [w2410]
            shift-right: [w2407] -> w2404
            shift-left: dbl[] [] -> [w2408]
            i -> [w2411]
            n981 = case shown="13" w2411 {
              tunnel: w2410 -> [w2412 w2423 w2434 w2444 w2454 w2464 w2476 w2488 w2500 w2512 w2524 w2536 w2550 w2572 w2584 w2593 w2602]
              tunnel: [w2413 w2424 w2435 w2445 w2455 w2466 w2478 w2490 w2502 w2514 w2526 w2537 w2559 w2575 w2583 w2592 w2604] -> w2409
              frame 0, Default {
                # "总电压过高"
                n982 = disable-structure shown="启用" {
                  disable-tunnel: [w2419 w2422] -> w2415
                  disable-tunnel: [w2418 w2422] -> w2414
                  disable-tunnel: w2412 -> [w2417 _]
                  frame Enabled {
                    n983 = Unbundle By Name(w2417) -> ("总电压过高"=w2416:dbl)
                    n984 = call "输入分辨率计算-EV05.vi"("1字节?"=FALSE, "数值"=w2416, "分辨率"=0.1) -> ("低字节"=w2419:dbl, "高字节1"=w2418:dbl)  [unwired: 2 in, 5 out]
                  }
                  frame Disabled {
                    w2422 = 255 ("高字节1")
                  }
                }
                n985 = Build Array(w2414, w2415) -> (w2413:dbl[])
              }
              frame 1 {
                # "总电压过低"
                n986 = disable-structure shown="启用" {
                  disable-tunnel: [w2430 w2433] -> w2426
                  disable-tunnel: [w2429 w2433] -> w2425
                  disable-tunnel: w2423 -> [w2428 _]
                  frame Disabled {
                    n987 = Unbundle By Name(w2428) -> ("总电压过低"=w2427:dbl)
                    n988 = call "输入分辨率计算-EV05.vi"("1字节?"=FALSE, "数值"=w2427, "分辨率"=0.1) -> ("低字节"=w2430:dbl, "高字节1"=w2429:dbl)  [unwired: 2 in, 5 out]
                  }
                  frame Enabled {
                    w2433 = 255 ("高字节1")
                  }
                }
                n989 = Build Array(w2425, w2426) -> (w2424:i32[])
              }
              frame 2 {
                # "温度过高"
                n990 = disable-structure shown="启用" {
                  disable-tunnel: [w2440 255 ("高字节1")] -> w2436
                  disable-tunnel: w2434 -> [w2438 _]
                  frame Disabled {
                    n991 = Unbundle By Name(w2438) -> ("温度过高"=w2437:dbl)
                    n992 = call "输入分辨率计算-EV05.vi"("1字节?"=TRUE, "数值"=w2437, "偏移量"=-40.0, "分辨率"=1.0) -> ("高字节1"=w2440:dbl)  [unwired: 1 in, 6 out]
                  }
                  frame Enabled {
                  }
                }
                n993 = Build Array(w2436) -> (w2435:i32[])
              }
              frame 3 {
                # "温度过低"
                n994 = disable-structure shown="启用" {
                  disable-tunnel: [w2450 255 ("高字节1")] -> w2446
                  disable-tunnel: w2444 -> [w2448 _]
                  frame Disabled {
                    n995 = Unbundle By Name(w2448) -> ("温度过低"=w2447:dbl)
                    n996 = call "输入分辨率计算-EV05.vi"("1字节?"=TRUE, "数值"=w2447, "偏移量"=-40.0, "分辨率"=1.0) -> ("高字节1"=w2450:dbl)  [unwired: 1 in, 6 out]
                  }
                  frame Enabled {
                  }
                }
                n997 = Build Array(w2446) -> (w2445:i32[])
              }
              frame 4 {
                # "整组温度不均衡"
                n998 = disable-structure shown="启用" {
                  disable-tunnel: [w2460 255 ("高字节1")] -> w2456
                  disable-tunnel: w2454 -> [w2458 _]
                  frame Disabled {
                    n999 = Unbundle By Name(w2458) -> ("整组温度不均衡"=w2457:dbl)
                    n1000 = call "输入分辨率计算-EV05.vi"("1字节?"=TRUE, "数值"=w2457, "偏移量"=0.0, "分辨率"=1.0) -> ("高字节1"=w2460:dbl)  [unwired: 1 in, 6 out]
                  }
